vi "PreparePath.vi"(10 "Numeric":i32, 11 "Path":path) -> (3 "appended path":path)   [LabVIEW 2016]
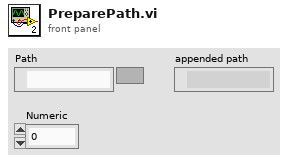
[diagram p1: front panel]
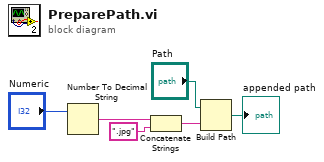
[diagram p0: block diagram]
diagram:
  n1 = Number To Decimal String(number="Numeric") -> (decimal integer string=w4:string)  [unwired: 1 in]
  n2 = Concatenate Strings(w4, ".jpg" ("string")) -> (w6:string)
  n3 = Build Path(base path="Path", name or relative path=w6) -> (appended path=→"appended path":path)
